vi "AddWriter.vi"(8 "Error in (no error)":errorcluster, 10 "LogWriterInterface in":refnum<class "LogWriterInterface.lvclass">, 11 "Log in":refnum<class "Log.lvclass">) -> (0 "Error out":errorcluster, 3 "Log out":refnum<class "Log.lvclass">)   [LabVIEW 2011, in "Log.lvclass"]
uses:
  Log.lvclass
  Writer/LogWriterInterface/LogWriterInterface.lvclass
  Log.lvclass/Log.ctl
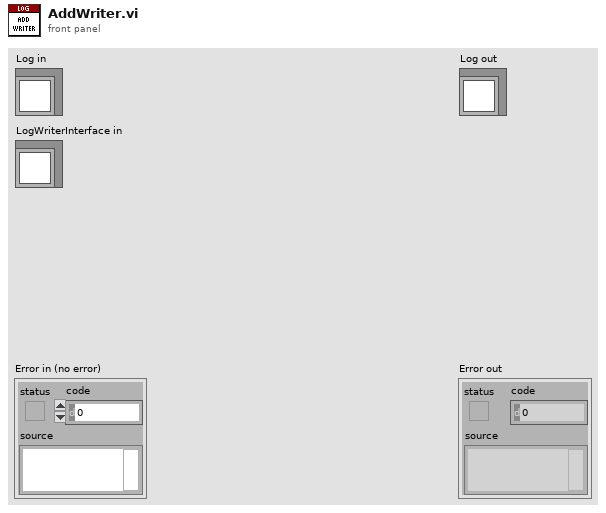
[diagram p1: front panel]
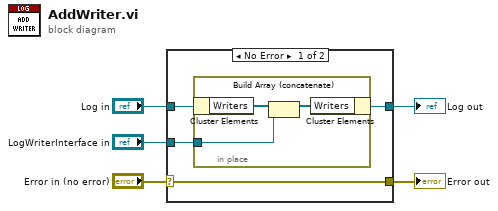
[diagram p0: block diagram]
diagram:
  n1 = case shown="No Error" "Error in (no error)" {
    selector: "Error in (no error)" -> [w9 w13]
    tunnel: [w9 w13] -> w4
    tunnel: [w7 w14] -> w2
    tunnel: "Log in" -> [w8 w14]
    tunnel: "LogWriterInterface in" -> [w6 _]
    frame No Error {
      n2 = in-place {
        in-place-border: w6 -> [w10]
        n3 = in-place-cluster #1(w8) -> ("Writers"=w12:refnum<class "LogWriterInterface.lvclass">[])
        n4 = Build Array (concatenate)(w12, w10) -> (w11:refnum<class "LogWriterInterface.lvclass">[])
        n5 = in-place-cluster #1("Writers"=w11) -> (w7:refnum<class "Log.lvclass">)
      }
    }
    frame Error {
    }
  }
  "Error out" <- w4
  "Log out" <- w2
